vi "Sixtypes Select.vi"() -> ()   [LabVIEW 2023]
doc: "This VI shows how you can read of different data types from a table named sixtypes in the LabVIEW.mdb database. \n\nThe table is created by the Sixtypes Insert VI, so it must be run before this VI in order to read data. Each of the values in the database table is a different data type and is converted by the Database Variant To Data function to their original LabVIEW data types."
uses:
  <vilib>/addons/database/Connection.llb/DB Tools Open Connec (Path).vi
  <vilib>/addons/database/_DB Variant To Data/Database Variant To Data.xnode
  <vilib>/addons/database/NI_Database_API.lvlib
panel:
  out "Date/Time":string
  out "Numeric (CDB)":cdb format="%.2f"
  out "Numeric (DBL)":dbl format="%#_6f"
  out "Numeric (SGL)":sgl format="%#_6f"
  out "Numeric (I32)":i32
  out "String":string
  # "Overview: Demonstrates how to read various data types from a table in a database.\nRequirements: Database Connectivity Toolkit\nInstructions:\n1. Make sure you have already run Sixtypes Insert.vi.\n2. Run the VI. All six data types are retrieved from the table."
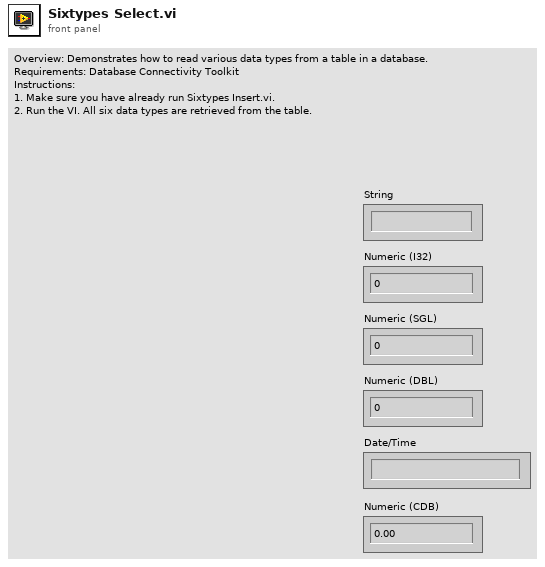
[diagram p1: front panel]
types:
  T1 = typedef "NI_Database_API.lvlib/Conn ObjectReference.ctl" = refnum<k1>
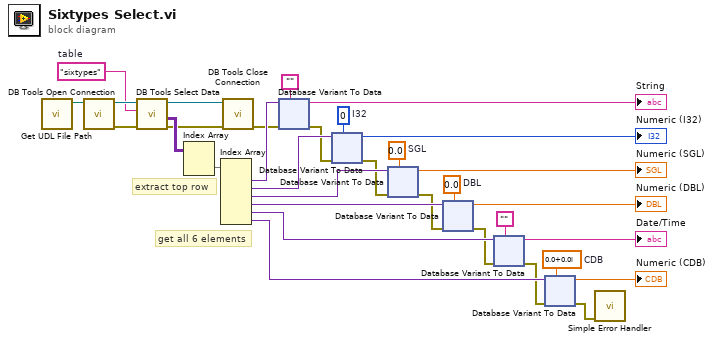
[diagram p0: block diagram]
diagram:
  w1 = cdb 0.0+0.0i  # CDB
  w3 = 0.0  # DBL
  w4 = sgl 0.0  # SGL
  w5 = 0  # I32
  w31 = "sixtypes"  # table
  # "get all 6 elements"
  # "extract top row"
  n1 = call "Get UDL File Path.vi"() -> ("UDL file path"=w6:path)  [unwired: 11 in]
  n2 = call-poly <vilib>:"DB Tools Open Connection.vi"("connection information"=w6) -> ("error out"=w33:errorcluster, "connection reference"=w32:T1)  [unwired: 7 in]
  n3 = call <vilib>:"DB Tools Select Data.vi"("error in (no error)"=w33, "table"=w31, "connection reference"=w32) -> ("error out"=w9:errorcluster, "data"=w17:variant[][], "connection reference out"=w10:T1)  [unwired: 3 in]
  n4 = Index Array(array=w17) -> (element=w18:variant[])  [unwired: 2 in]
  n5 = Index Array(array=w18) -> (element #1=w30:variant, element #2=w29:variant, element #3=w28:variant, element #4=w27:variant, element #5=w26:variant, element #6=w25:variant)  [unwired: 6 in]
  n6 = call <vilib>:"DB Tools Close Connection.vi"("error in (no error)"=w9, "connection reference"=w10) -> ("error out"=w8:errorcluster)  [unwired: 5 in]
  n7 = xnode "Database Variant To Data"("database variant"=w30, "error in (no error)"=w8, "type"="" ("String")) -> ("data"=→"String":string, "error out"=w24:errorcluster)
  n8 = xnode "Database Variant To Data"("database variant"=w29, "error in (no error)"=w24, "type"=w5) -> ("data"=→"Numeric (I32)":i32, "error out"=w23:errorcluster)
  n9 = xnode "Database Variant To Data"("database variant"=w28, "error in (no error)"=w23, "type"=w4) -> ("data"=→"Numeric (SGL)":sgl, "error out"=w22:errorcluster)
  n10 = xnode "Database Variant To Data"("database variant"=w27, "error in (no error)"=w22, "type"=w3) -> ("data"=→"Numeric (DBL)":dbl, "error out"=w21:errorcluster)
  n11 = xnode "Database Variant To Data"("database variant"=w26, "error in (no error)"=w21, "type"="") -> ("data"=→"Date/Time":string, "error out"=w20:errorcluster)
  n12 = xnode "Database Variant To Data"("database variant"=w25, "error in (no error)"=w20, "type"=w1) -> ("data"=→"Numeric (CDB)":cdb, "error out"=w7:errorcluster)
  n13 = call <vilib>:"Simple Error Handler.vi"("error in (no error)"=w7) -> ()  [unwired: 4 in, 5 out]
